vi "Calibration.vi"() -> ()   [LabVIEW 2021]
uses:
  <vilib>/Platform/TimedLoop/XDataNode/timing_clust.ctl
  <vilib>/Platform/TimedLoop/XDataNode/nitl_modes.ctl
  <vilib>/Platform/TimedLoop/XDataNode/wakeup.ctl
  <vilib>/platform/TimedLoop/XDataNode/XDataNode.xnode
  <vilib>/Platform/TimedLoop/XDataNode/XDNodeRunTimeDep.lvlib
panel:
  in  "file path (trajectorymat)":path=path "c:/ni-rt/startup/trajectorymat_asta0_line.csv"
  in  "file path (matrixmat)":path=path "c:/ni-rt/startup/matrixmat_default.csv"
  out "Gyroscope Bias (rad/s)":T1
  in  "Calibration Time (s)":dbl=5.0
  in  "Sampling Period (us)":i64=10000
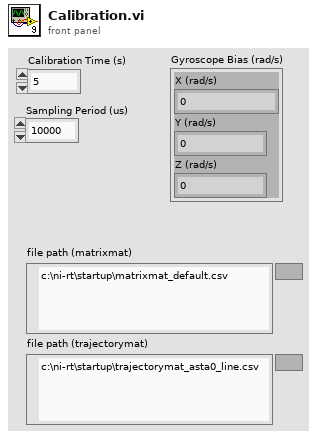
[diagram p1: front panel]
types:
  T1 = cluster{"X (rad/s)":dbl, "Y (rad/s)":dbl, "Z (rad/s)":dbl}
  T2 = typedef "Configuration.ctl" = cluster{"Accelerometer Bias":cluster{"X (m/s)":dbl, "Y (m/s)":dbl, "Z (m/s)":dbl}, "Gyroscope Bias":cluster{"X (m/s)":dbl, "Y (m/s)":dbl, "Z (m/s)":dbl}, "Steering Motor Gear Ratio":dbl, "Steering Pully Gear Ratio":dbl, "Steering Encoder CPR":dbl, "Steering Motor Max RPM":dbl, "Wheelbase (m)":dbl, "Fork Angle (rad)":dbl, "Balancing Controller":cluster{"Kp (/s)":dbl, "Kd (1)":dbl}, "Max Allowed Steering Angle (rad)":dbl, "Task Periods":cluster{"Emergency Stop (us)":i64, "IMU (us)":i64, "Steering Motor Encoder (us)":i64, "State Estimator (us)":i64, "Balancing Controller (us)":i64, "GNSS (us)":i64, "Logging (us)":i64, "Drive Motor (us)":i64, "Visualization (us)":i64}, "Drive Motor Gear Ratio":dbl, "lr":dbl, "lf":dbl, "lambda":dbl, "k1":dbl, "k2":dbl, "e1_max":dbl, "Ad_t":dbl, "Bd_t":dbl, "C_t":dbl, "D_t":dbl, "Wheel radius":dbl}
  T3 = typedef "XDNodeRunTimeDep.lvlib/timing_clust.ctl" = cluster{"Expected End [f-1]":u64, "Actual End [f-1]":u64, "Finished Late? [f-1]":bool, "Expected End [i-1]":u64, "Actual End [i-1]":u64, "Finished Late? [i-1]":bool, "Expected Start [i]":u64, "Actual Start [i]":u64, "Expected Start [f]":u64, "Actual Start [f]":u64, "Source Name":string, "Structure Name":string, "Period":i64, "Deadline":i64, "Offset":i64, "Start":i64, "Priority":i32, "Timeout":i32, "Mode":T4, "Wakeup Reason":T5, "Error":errorcluster, "Source Type":string, "Secondary Source Type":string, "Global End Time":u64, "Global Start Time":u64, "Frame Duration":u64, "Iteration Duration":u64, "Assigned CPU":i32, "I/O Scan Engine Mode":u32}
  T4 = typedef "XDNodeRunTimeDep.lvlib/nitl_modes.ctl" = enum32{"No Change", "Process missed periods, maintain original phase", "Discard missed periods, maintain original phase", "Process missed periods, ignore original phase", "Discard missed periods, ignore original phase"}
  T5 = typedef "XDNodeRunTimeDep.lvlib/wakeup.ctl" = enum32{"Normal", "Aborted", "Asynchronous wakeup", "Timing source error", "Timed loop error", "Timeout"}
  T6 = typedef "IMU Handle.ctl" = cluster{"I2C address":u8}
  T7 = typedef "IMU Data.ctl" = cluster{"Gyroscope":cluster{"X (rad/s)":dbl, "Y (rad/s)":dbl, "Z (rad/s)":dbl}, "Accelerometer":cluster{"X (m/s^2)":dbl, "Y (m/s^2)":dbl, "Z (m/s^2)":dbl}, "Flag IMU":dbl}
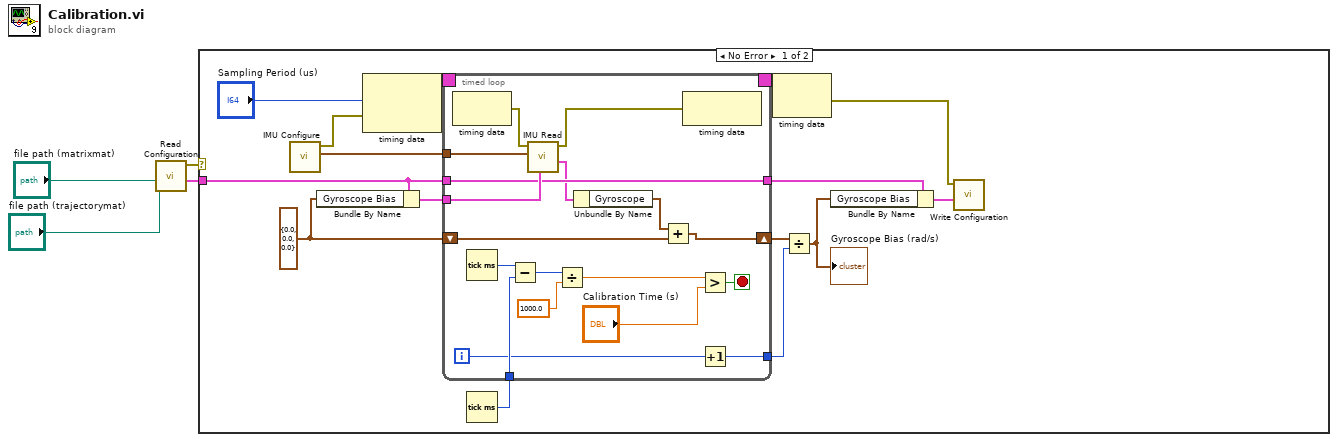
[diagram p0: block diagram]
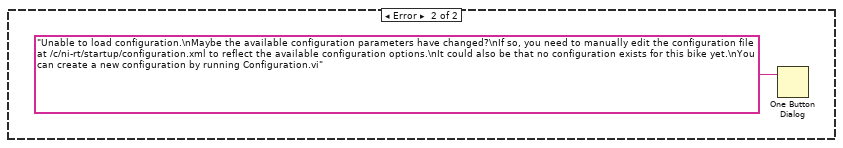
[diagram p2: hidden frame]
diagram:
  n1 = call "Read Configuration.vi"("file path (trajectorymat)"="file path (trajectorymat)", "file path (matrixmat)"="file path (matrixmat)") -> ("configuration"=w3:T2, "error out"=w4:errorcluster)  [unwired: 3 in, 5 out]
  n2 = case shown="No Error" w4 {
    tunnel: w3 -> [w11 _]
    frame No Error {
      w7 = T1 {"X (rad/s)"=0.0, "Y (rad/s)"=0.0, "Z (rad/s)"=0.0}
      n3 = call "IMU Configure.vi"() -> ("IMU Handle"=w14:T6, "Error Out"=w15:errorcluster)  [unwired: 10 in]
      n4 = Bundle By Name(cluster=w11, "Gyroscope Bias"=w7) -> (w12:T2)
      n5 = node-c288("Sampling Period (us)", w15) -> (w19:T3)
      n6 = Tick Count (ms)() -> (millisecond timer value=w16:u32)
      n7 = timed-loop {
        timing: w19 -> [_]
        timing-out: [_] -> w18
        tunnel: w16 -> [w36]
        tunnel: w14 -> [w30]
        shift-right: [w21] -> w6
        shift-left: w7 -> [w20]
        tunnel: [w26] -> w13
        tunnel: w12 -> [w25]
        tunnel: w11 -> [w24]
        tunnel: [w24] -> w10
        i -> [w27]
        stop <- w31 stop-if-true
        n8 = node-c288() -> (w29:errorcluster)  [unwired: 1 in]
        n9 = Tick Count (ms)() -> (millisecond timer value=w37:u32)
        n10 = Subtract(x=w37, y=w36) -> (x-y=w35:u32)
        n11 = call "IMU Read.vi"("Configuration"=w25, "IMU Handle"=w30, "Error In"=w29) -> ("IMU Data"=w23:T7, "Error Out"=w28:errorcluster)  [unwired: 6 in, 1 out]
        n12 = Divide(x=w35, y=1000.0) -> (x/y=w33:dbl)
        n13 = Unbundle By Name(w23) -> ("Gyroscope"=w22:T1)
        n14 = Add(x=w22, y=w20) -> (x+y=w21:T1)
        n15 = node-c288(w28) -> ()  [unwired: 1 out]
        n16 = Greater?(x=w33, y="Calibration Time (s)") -> (0:w31:bool)
        n17 = Increment(x=w27) -> (x+1=w26:i32)
      }
      n18 = node-c288(w18) -> (w8:errorcluster)
      n19 = Divide(x=w6, y=w13) -> (x/y=w5:T1)
      "Gyroscope Bias (rad/s)" <- w5
      n20 = Bundle By Name(cluster=w10, "Gyroscope Bias"=w5) -> (w9:T2)
      n21 = call "Write Configuration.vi"("Configuration"=w9, "Error In"=w8) -> ()  [unwired: 9 in, 1 out]
    }
    frame Error {
      n22 = One Button Dialog(message="Unable to load configuration.\nMaybe the available configuration parameters have changed?\nIf so, you need to manually edit the configuration file at /c/ni-rt/startup/configuration.xml to reflect the available configuration options.\nIt could also be that no configuration exists for this bike yet.\nYou can create a new configuration by running Configuration.vi") -> ()  [unwired: 1 in, 1 out]
    }
  }
